vi "Begin.vi"(8 "error in":errorcluster) -> (0 "error out":errorcluster)   [LabVIEW 2016]
doc: "Called before other user functions, this VI is expected to open initial I/O refnums, load in file data, and do all program initialization. Notice that the <B>error out</B> terminal is simply used for data flow. Wiring it to other structures or subVIs ensures that this VI runs first."
uses:
  <vilib>/Rock Robotics/WPI/DriverStation/WPI_DriverStationRobotMode2.ctl
  <vilib>/Rock Robotics/WPI/Joystick/WPI_JoystickDeviceEnum.ctl
  <vilib>/Rock Robotics/SystemInterfaces/DIO/FPGA_DIOChannel.ctl
  <vilib>/Rock Robotics/SystemInterfaces/spilib/spi_bus.ctl
  <vilib>/Rock Robotics/SystemInterfaces/DIO/FPGA_DIORelayChannel.ctl
  <vilib>/Rock Robotics/WPI/Relay/WPI_RelayDirection.ctl
  <vilib>/Rock Robotics/WPI/ThirdParty/CanMotor/TalonSRX/WPI_CANTalonSRX_APIControlMode.ctl
  <vilib>/Rock Robotics/WPI/ThirdParty/CanMotor/TalonSRX/WPI_CANTalonSRX_APIFeedbackSelect.ctl
  Robot Global Data.vi
  <vilib>/Rock Robotics/Network Tables/NT Write String Array.vi
  <vilib>/Rock Robotics/WPI/Ultrasonic/WPI_SonarMB1010DigitalOpen.vi
  <vilib>/Rock Robotics/WPI/Ultrasonic/WPI_SonarMB1010DigRefNum Registry Set.vi
  <vilib>/Rock Robotics/WPI/Gyro/WPI_GyroXRS450_SPI_Open.vi
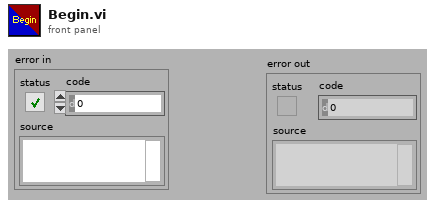
[diagram p1: front panel]
types:
  T1 = typedef "WPI_CANTalonSRX_APIFeedbackSelect.ctl" = enum16{"Digital Quadrature Encoder", "Analog Potentiometer", "Analog Encoder", "Count on Quad-A (Rising-Edge)", "Count on Quad-A (Falling-Edge)", "CTR Magnetic Enc (Absolute)", "CTR Magnetic Enc (Relative)", "Pulse Width"}
  T2 = typedef "WPI_CANTalonSRX_APIControlMode.ctl" = enum8{"Percent VBus", "Speed", "Position", "Slave", "Unchanged / Invalid", "Voltage Compensation", "Current", "Motion Profile", "Motion Magic"}
  T3 = typedef "WPI_RelayDirection.ctl" = enum16{"Both directions", "Forward only", "Reverse only"}
  T4 = typedef "FPGA_DIORelayChannel.ctl" = enum8{"Relay 0", "Relay 1", "Relay 2", "Relay 3", "Invalid"}
  T5 = typedef "spi_bus.ctl" = enum16{"SPI On-Board, CS0", "SPI On-Board, CS1", "SPI On-Board, CS2", "SPI On-Board, CS3", "SPI MXP", "Invalid"}
  T6 = typedef "WPI_JoystickDeviceEnum.ctl" = enum16{"USB 0", "USB 1", "USB 2", "USB 3", "USB 4", "USB 5"}
  T7 = typedef "FPGA_DIOChannel.ctl" = enum8{"DIO 0", "DIO 1", "DIO 2", "DIO 3", "DIO 4", "DIO 5", "DIO 6", "DIO 7", "DIO 8", "DIO 9", "DIO MXP 0", "DIO MXP 1", "DIO MXP 2", "DIO MXP 3", "DIO MXP 4", "DIO MXP 5", "DIO MXP 6", "DIO MXP 7", "DIO MXP 8", "DIO MXP 9", "DIO MXP 10", "DIO MXP 11", "DIO MXP 12", "DIO MXP 13", "DIO MXP 14", "DIO MXP 15", "SPI Port CS1", "SPI Port CS2", "SPI Port CS3", "SPI Port MISO", "SPI Port MOSI", "Invalid"}
  T8 = typedef "WPI_DriverStationRobotMode2.ctl" = enum16{"Autonomous Disabled", "Autonomous Enabled", "Teleop Disabled", "Teleop Enabled", "Disconnected", "Finish", "Test Disabled", "Test Enabled", "Emergency Stopped"}
  T9 = typedef "WPI_MotorControlDeviceRef.ctl" = cluster{"DeviceStatus":errorcluster, "Type":T10, "PWM":cluster{"PWM Channel":T11, "DeadBand":T12}, "CAN":cluster{"Device Number":u8, "SetOutput VI Ref":variant, "GetOutput VI Ref":variant, "Enable VI Ref":variant, "Disable VI Ref":variant, "Data":variant}, "Invert":bool}
  T10 = typedef "WPI_MotorControlType.ctl" = enum16{"PWM", "CAN"}
  T11 = typedef "FPGA_DIOPWMChannel.ctl" = enum8{"PWM 0", "PWM 1", "PWM 2", "PWM 3", "PWM 4", "PWM 5", "PWM 6", "PWM 7", "PWM 8", "PWM 9", "PWM MXP 0", "PWM MXP 1", "PWM MXP 2", "PWM MXP 3", "PWM MXP 4", "PWM MXP 5", "PWM MXP 6", "PWM MXP 7", "PWM MXP 8", "PWM MXP 9", "Invalid"}
  T12 = typedef "WPI_PWMDeadband.ctl" = cluster{"Name":string, "maxPositivePwm":i32, "minPositivePwm":i32, "centerPwm":i32, "maxNegativePwm":i32, "minNegativePwm":i32, "angularRange":u16}
  T13 = typedef "WPI_JoystickDevRef.ctl" = cluster{"Device":T6}
  T14 = typedef "WPI_SonarMB1010DigitalDeviceRef.ctl" = cluster{"CounterDevRef":T15, "Scaling factor (s/in)":dbl}
  T15 = typedef "WPI_CounterDevRef.ctl" = cluster{"DevStatus":errorcluster, "CntIndex":T16}
  T16 = typedef "FPGA_CounterCtrSystemIndex.ctl" = enum8{"Ctr 0", "Ctr 1", "Ctr 2", "Ctr 3", "Ctr 4", "Ctr 5", "Ctr 6", "Ctr 7", "Invalid"}
  T17 = typedef "WPI_RelayDevRef.ctl" = cluster{"DevStatus":errorcluster, "Relay Channel":T4, "Relay Direction":T3}
  T18 = typedef "WPI_GyroDevRef.ctl" = cluster{"DevStatus":errorcluster, "Analog Channel":T19, "Offset":dbl, "Gain (VoltsPerDegree/Second)":dbl, "Gyro Type":enum16{"Analog", "XRS450"}, "Handle":i32, "SPI Bus":T5, "Device Found":bool, "Sample Rate":dbl, "Calibrate On Open":bool}
  T19 = typedef "FPGA_AIChannel.ctl" = enum8{"AI 0", "AI 1", "AI 2", "AI 3", "AI MXP 0", "AI MXP 1", "AI MXP 2", "AI MXP 3", "Invalid"}
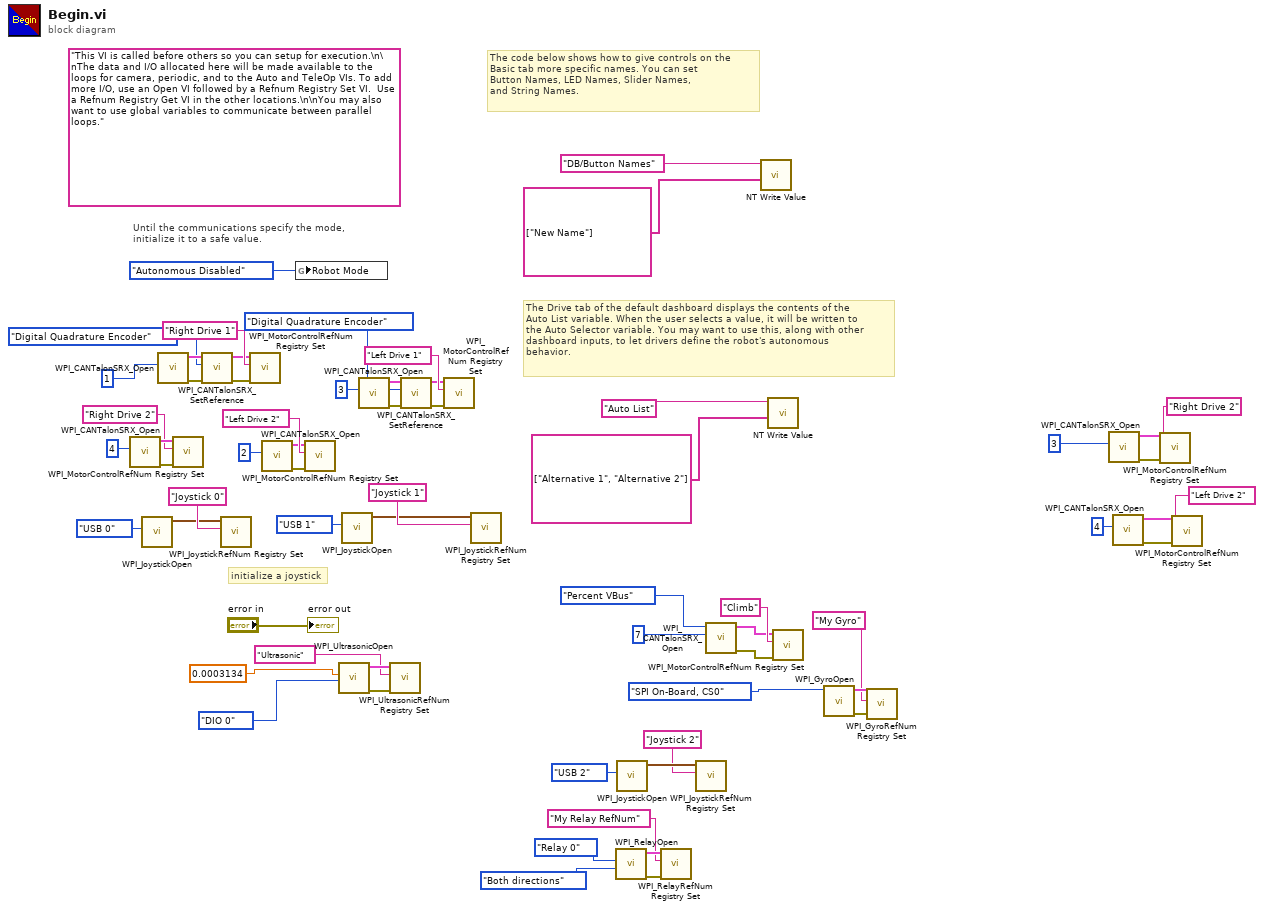
[diagram p0: block diagram]
diagram:
  (unwired) "This VI is called before others so you can setup for execution.\n\nThe data and I/O allocated here will be made available to the loops for camera, periodic, and to the Auto and TeleOp VIs. To add more I/O, use an Open VI followed by a Refnum Registry Set VI.  Use a Refnum Registry Get VI in the other locations.\n\nYou may also want to use global variables to communicate between parallel loops."
  # "The Drive tab of the default dashboard displays the contents of the\nAuto List variable. When the user selects a value, it will be written to\nthe Auto Selector variable. You may want to use this, along with other\ndashboard inputs, to let drivers define the robot's autonomous\nbehavior."
  # "The code below shows how to give controls on the\nBasic tab more specific names. You can set\nButton Names, LED Names, Slider Names,\nand String Names."
  # "initialize a joystick"
  # "Until the communications specify the mode,\ninitialize it to a safe value."
  n1 = call <vilib>:"WPI_CANTalonSRX_Open.vi"("Device Number"=u8 4) -> ("error out"=w13:errorcluster, "CAN Talon SRX Ref"=w14:T9)  [unwired: 9 in]
  n2 = call <vilib>:"WPI_JoystickOpen.vi"("JoystickDevice"=WPI_JoystickDeviceEnum."USB 0") -> ("JoystickDevRef"=w62:T13)  [unwired: 10 in]
  n3 = call <vilib>:"WPI_CANTalonSRX_Open.vi"("Device Number"=u8 1) -> ("error out"=w5:errorcluster, "CAN Talon SRX Ref"=w6:T9)  [unwired: 9 in]
  n4 = call <vilib>:"WPI_MotorControlRefNum Registry Set.vi"("error in (no error)"=w13, "refnum name"="Right Drive 2", "MotorControlDevRef"=w14) -> ()  [unwired: 7 in, 2 out]
  n5 = call <vilib>:"WPI_CANTalonSRX_SetReference.vi"("error in (no error)"=w5, "Feedback Reference"=WPI_CANTalonSRX_APIFeedbackSelect."Digital Quadrature Encoder", "CAN Talon SRX Ref"=w6) -> ("error out"=w4:errorcluster, "CAN Talon SRX Ref"=w3:T9)  [unwired: 7 in]
  n6 = call <vilib>:"WPI_JoystickRefNum Registry Set.vi"("refnum name"="Joystick 0", "JoystickDevRef"=w62) -> ()  [unwired: 8 in, 2 out]
  n7 = call <vilib>:"WPI_MotorControlRefNum Registry Set.vi"("error in (no error)"=w4, "refnum name"="Right Drive 1", "MotorControlDevRef"=w3) -> ()  [unwired: 7 in, 2 out]
  n8 = call <vilib>:"WPI_CANTalonSRX_Open.vi"("Device Number"=u8 2) -> ("error out"=w16:errorcluster, "CAN Talon SRX Ref"=w15:T9)  [unwired: 9 in]
  n9 = global write "Robot Global Data.vi" "Robot Mode"(WPI_DriverStationRobotMode2."Autonomous Disabled" ("Robot Mode")) -> ()
  n10 = call <vilib>:"WPI_MotorControlRefNum Registry Set.vi"("error in (no error)"=w16, "refnum name"="Left Drive 2", "MotorControlDevRef"=w15) -> ()  [unwired: 7 in, 2 out]
  n11 = call-poly <vilib>:"WPI_UltrasonicOpen.vi"("Scaling factor (s/in)"=0.0003134, "DIO Channel"=FPGA_DIOChannel."DIO 0") -> ("error out"=w48:errorcluster, "SonarMB1010DigitalDevRef"=w47:T14)  [unwired: 8 in]
  n12 = call <vilib>:"WPI_JoystickOpen.vi"("JoystickDevice"=WPI_JoystickDeviceEnum."USB 1") -> ("JoystickDevRef"=w54:T13)  [unwired: 10 in]
  n13 = call <vilib>:"WPI_CANTalonSRX_Open.vi"("Device Number"=u8 3) -> ("error out"=w10:errorcluster, "CAN Talon SRX Ref"=w9:T9)  [unwired: 9 in]
  n14 = call-poly <vilib>:"WPI_UltrasonicRefNum Registry Set.vi"("error in (no error)"=w48, "refnum name"="Ultrasonic", "SonarMB1010DigitalDevRef"=w47) -> ()  [unwired: 7 in, 2 out]
  n15 = call <vilib>:"WPI_CANTalonSRX_SetReference.vi"("error in (no error)"=w10, "Feedback Reference"=WPI_CANTalonSRX_APIFeedbackSelect."Digital Quadrature Encoder", "CAN Talon SRX Ref"=w9) -> ("error out"=w7:errorcluster, "CAN Talon SRX Ref"=w8:T9)  [unwired: 7 in]
  n16 = call <vilib>:"WPI_MotorControlRefNum Registry Set.vi"("error in (no error)"=w7, "refnum name"="Left Drive 1", "MotorControlDevRef"=w8) -> ()  [unwired: 7 in, 2 out]
  n17 = call <vilib>:"WPI_JoystickRefNum Registry Set.vi"("refnum name"="Joystick 1", "JoystickDevRef"=w54) -> ()  [unwired: 8 in, 2 out]
  n18 = call <vilib>:"WPI_RelayOpen.vi"("Relay Direction"=WPI_RelayDirection."Both directions", "Relay Channel"=FPGA_DIORelayChannel."Relay 0") -> ("error out"=w35:errorcluster, "RelayDevRef"=w34:T17)  [unwired: 8 in]
  n19 = call <vilib>:"WPI_JoystickOpen.vi"("JoystickDevice"=WPI_JoystickDeviceEnum."USB 2") -> ("JoystickDevRef"=w42:T13)  [unwired: 10 in]
  n20 = call <vilib>:"WPI_RelayRefNum Registry Set.vi"("error in (no error)"=w35, "refnum name"="My Relay RefNum", "RelayDevRef"=w34) -> ()  [unwired: 7 in, 2 out]
  n21 = call <vilib>:"WPI_JoystickRefNum Registry Set.vi"("refnum name"="Joystick 2", "JoystickDevRef"=w42) -> ()  [unwired: 8 in, 2 out]
  n22 = call <vilib>:"WPI_CANTalonSRX_Open.vi"("Device Number"=u8 7, "Control Mode"=WPI_CANTalonSRX_APIControlMode."Percent VBus") -> ("error out"=w27:errorcluster, "CAN Talon SRX Ref"=w28:T9)  [unwired: 8 in]
  n23 = call-poly <vilib>:"NT Write Value.vi"("String Array"=string[] ["New Name"], "Name"="DB/Button Names") -> ()  [unwired: 9 in, 1 out]
  n24 = call-poly <vilib>:"NT Write Value.vi"("String Array"=string[] ["Alternative 1", "Alternative 2"], "Name"="Auto List") -> ()  [unwired: 9 in, 1 out]
  n25 = call <vilib>:"WPI_MotorControlRefNum Registry Set.vi"("error in (no error)"=w27, "refnum name"="Climb", "MotorControlDevRef"=w28) -> ()  [unwired: 7 in, 2 out]
  n26 = call-poly <vilib>:"WPI_GyroOpen.vi"("SPI Bus"=spi_bus."SPI On-Board, CS0") -> ("error out"=w39:errorcluster, "GyroDevRef"=w38:T18)  [unwired: 9 in]
  n27 = call <vilib>:"WPI_GyroRefNum Registry Set.vi"("error in (no error)"=w39, "refnum name"="My Gyro", "GyroDevRef"=w38) -> ()  [unwired: 7 in, 2 out]
  n28 = call <vilib>:"WPI_CANTalonSRX_Open.vi"("Device Number"=u8 3) -> ("error out"=w26:errorcluster, "CAN Talon SRX Ref"=w25:T9)  [unwired: 9 in]
  n29 = call <vilib>:"WPI_CANTalonSRX_Open.vi"("Device Number"=u8 4) -> ("error out"=w24:errorcluster, "CAN Talon SRX Ref"=w23:T9)  [unwired: 9 in]
  n30 = call <vilib>:"WPI_MotorControlRefNum Registry Set.vi"("error in (no error)"=w26, "refnum name"="Right Drive 2", "MotorControlDevRef"=w25) -> ()  [unwired: 7 in, 2 out]
  n31 = call <vilib>:"WPI_MotorControlRefNum Registry Set.vi"("error in (no error)"=w24, "refnum name"="Left Drive 2", "MotorControlDevRef"=w23) -> ()  [unwired: 7 in, 2 out]
  "error out" <- "error in"
